vi "ENUM Array_To String Array.vi"(4 "ENUM Array":variant[](array[variant])) -> (1 "String Array Out":string[](array[string]))   [LabVIEW 2015]
uses:
  <vilib>/Utility/VariantDataType/VariantType.lvlib
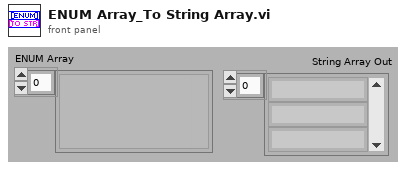
[diagram p1: front panel]
types:
  T1 = typedef "VariantType.lvlib/Type.ctl" = enum8{"Invalid Type", "Void", "I8", "I16", "I32", "I64", "U8", "U16", "U32", "U64", "Single Float", "Double Float", "Extended Float", "Single Complex", "Double Complex", "Extended Complex", "Enum U8", "Enum U16", "Enum U32", "Enum U64", "Single Float With Unit", "Double Float With Unit", "Extended Float With Unit", "Single Complex with Unit", "Double Complex with Unit", "Extended Complex with Unit", "Boolean", "String", "Path", "Picture", "Tag", "Array", "Cluster", "Variant", "LV Variant", "Waveform", "Timestamp", "Digital Waveform", "Digital Data", "ExpressData", "Refnum", "External Data", "VI", "Poly VI", "LabVIEW Class Instance", "Fixed Point"}
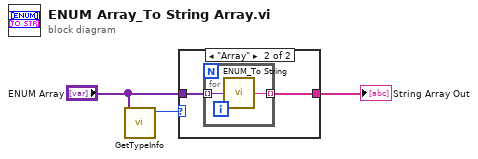
[diagram p0: block diagram]
diagram:
  n1 = call <vilib>:"GetTypeInfo.vi"("Variant"="ENUM Array") -> ("Type Enum"=w1:T1)  [unwired: 6 in, 4 out]
  n2 = case shown="\"Array\"" w1 {
    tunnel: [_ w5] -> w3
    tunnel: "ENUM Array" -> [_ w4]
    frame Default {
    }
    frame "Array" {
      n3 = for {
        tunnel: w4 -> [w7] mode=indexing
        tunnel: [w6] -> w5 mode=indexing
        n4 = call "ENUM_To String.vi"("ENUM"=w7) -> ("String Out"=w6:string)  [unwired: 4 in]
      }
    }
  }
  "String Array Out" <- w3
